vi "Memory.Pointer.Check.vi"(8 "error in (no error)":errorcluster, 11 "pointer in":refnum<class "Memory.Pointer.lvclass">) -> (0 "error out":errorcluster, 2 "LabVIEW pointer?":bool, 3 "pointer out":refnum<class "Memory.Pointer.lvclass">)   [LabVIEW 2016, in "Memory Manager.lvlib" / "Memory.Pointer.lvclass"]
doc: "Checks that the provided <b>pointer</b> was allocated by LabVIEW."
uses:
  Memory.Pointer.lvclass
  Memory.Pointer.lvclass/Memory.Pointer.ctl
  Memory.Pointer.Errors.vi
  Memory.Pointer.Errors.Null Pointer.vi
  Memory.Pointer.Errors.Create Error.vi
  Submodules/Static Error Handling/Source/Library/VIs/Static Error Handling.Error Cluster Constant.vi
  Submodules/Static Error Handling/Source/Library/VIs/Static Error Handling.Error Cluster Constant (256B).vi
  Submodules/Static Error Handling/Source/Library/VIs/Static Error Handling.Parameters.Status.Set.vi
  Submodules/Static Error Handling/Source/Library/VIs/Static Error Handling.Parameters.Code.Set.vi
  Submodules/Static Error Handling/Source/Library/VIs/Static Error Handling.Parameters.VI Source.Set.vi
  Constants/Memory.Constants.vi
  Constants/Memory.Constants.Library Name.vi
  Memory.Pointer.Errors.Get Info.vi
  Submodules/Static Error Handling/Source/Library/VIs/Static Error Handling.Source Buffer.Write.String.vi
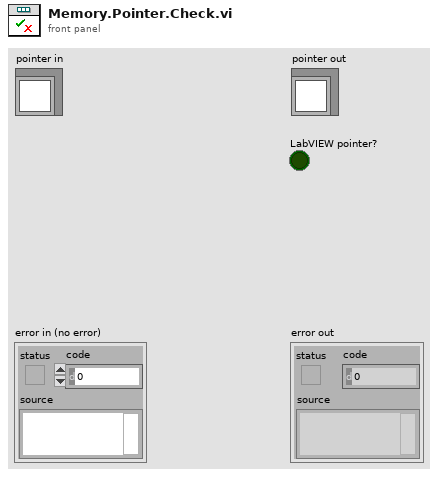
[diagram p1: front panel]
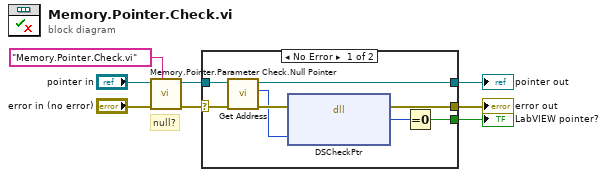
[diagram p0: block diagram]
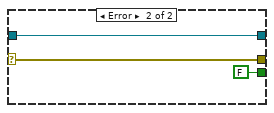
[diagram p2: hidden frame]
diagram:
  # "null?"
  n1 = call "Memory.Pointer.Parameter Check.Null Pointer.vi"("source vi name"="Memory.Pointer.Check.vi", "error in (no error)"="error in (no error)", "Pointer in"="pointer in") -> ("error out"=w1:errorcluster, "Pointer out"=w3:refnum<class "Memory.Pointer.lvclass">)  [unwired: 7 in]
  n2 = case shown="No Error" w1 {
    selector: w1 -> [w9 w18]
    tunnel: [w16 w19] -> w8
    tunnel: [w13 w18] -> w7
    tunnel: [w11 FALSE] -> w6
    tunnel: w3 -> [w10 w19]
    frame No Error {
      n3 = call "Get Address.vi"("error in (no error)"=w9, "Pointer in"=w10) -> ("error out"=w15:errorcluster, "address"=w14:u64, "Pointer out"=w16:refnum<class "Memory.Pointer.lvclass">)  [unwired: 7 in]
      n4 = dll-call lib="LabVIEW" fn="DSCheckPtr"(error in=w15, "pointer"=w14) -> (error out=w13:errorcluster, "return"=w12:i32)  [unwired: 3 in, 1 out]
      n5 = Equal To 0?(x=w12) -> (x = 0?=w11:bool)
    }
    frame Error {
    }
  }
  "error out" <- w7
  "pointer out" <- w8
  "LabVIEW pointer?" <- w6
